vi "mod_Truncate Filter Transient.vi"(9 "filter length (sym)":i32, 10 "samples/symbol":i32, 11 "input complex waveform":T1={"t0"=0.0, "dt"=1.0, "Y"=[]} {"Y" format="%.3f"; "dt" format="%^.2e"; "t0" format="%.4f"}) -> (3 "output complex waveform":T1={"t0"=0.0, "dt"=1.0, "Y"=[]} {"Y" format="%.3f"; "dt" format="%^.2e"; "t0" format="%.4f"})   [LabVIEW 2020, in "niDMT.lvlib"]
uses:
  <vilib>/addons/Modulation/niDMT.lvlib
  <vilib>/addons/Modulation/Analog/controls/Complex Data Waveform.ctl
  <vilib>/addons/Modulation/niAMT.lvlib
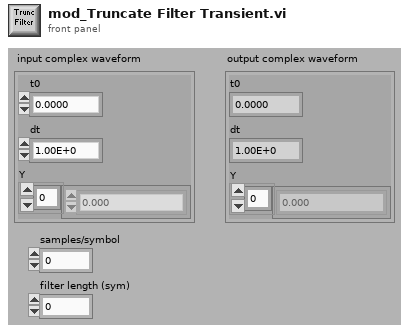
[diagram p1: front panel]
types:
  T1 = typedef "niAMT.lvlib/Complex Data Waveform.ctl" = cluster{"t0":dbl, "dt":dbl, "Y":cdb[]}
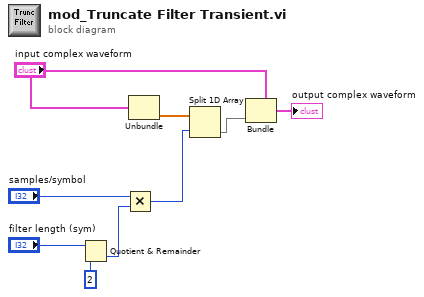
[diagram p0: block diagram]
diagram:
  n1 = Quotient & Remainder(x="filter length (sym)", y=2) -> (floor(x/y)=w2:i32)  [unwired: 1 out]
  n2 = Multiply(x="samples/symbol", y=w2) -> (x*y=w1:i32)
  n3 = Unbundle("input complex waveform") -> ("Y"=w7:cdb[])  [unwired: 2 out]
  n4 = Split 1D Array(array=w7, index=w1) -> (second subarray=w4:cdb[])  [unwired: 1 out]
  n5 = Bundle(cluster="input complex waveform", "Y"=w4) -> (→"output complex waveform":T1)  [unwired: 2 out]
